vi "WSS.Generate.Digital.vi"(11 "Settings":T1={"ACTIVE EDGE"=TRUE, "ACTIVE TICKS"=0, "INACTIVE TICKS"=0, "DATA"=0, "SENSOR TYPE"=0}) -> (1 "Bit1":bool, 2 "Bit0":bool, 3 "Pulse":bool)   [LabVIEW 2018, in "Speciality FPGA IO.lvlib"]
doc: "This VI Simulates Wheel Speed Sensors for Unidirectional, Bidirectional - Bosch, and Bidirectional Conti. Sensor Type is:\n0 - Unidirectional\n1 - Bidirectional Bosch\n2 - Bidirectional Continental. The output of the VI is two digital bits that correspond to the following current levels when paired with an OW-902 module:\nBit 0 Bit 1 Output Current Level\n0 0 0\n0 1 Lo\n1 0 Mid\n1 1 Hi"
uses:
  <vilib>/NI/FPGA Addon Specialty IO/Speciality FPGA IO.lvlib
  <vilib>/NI/FPGA Addon Specialty IO/Types/WSS.Generate.Digital.Settings.ctl
  <vilib>/NI/FPGA Addon Specialty IO/Types/PWM.Generate.Digital.Settings.ctl
  <vilib>/NI/FPGA Addon Specialty IO/Types/WSS.Sensor.Type.ctl
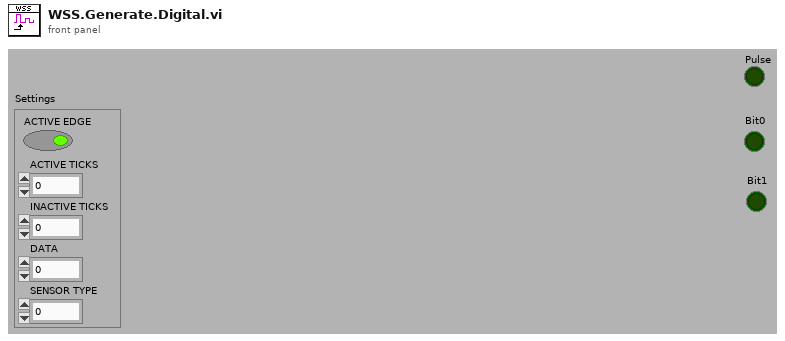
[diagram p1: front panel]
types:
  T1 = typedef "Speciality FPGA IO.lvlib/WSS.Generate.Digital.Settings.ctl" = cluster{"ACTIVE EDGE":bool, "ACTIVE TICKS":u32, "INACTIVE TICKS":u32, "DATA":u8, "SENSOR TYPE":u8}
  T2 = typedef "Speciality FPGA IO.lvlib/PWM.Generate.Digital.Settings.ctl" = cluster{"ACTIVE EDGE":bool, "ACTIVE TICKS":u32, "INACTIVE TICKS":u32}
  T3 = typedef "Speciality FPGA IO.lvlib/WSS.Sensor.Type.ctl" = enum16{"Unidirectional", "Bosch Bidirectional", "Continental Bidirectional"}
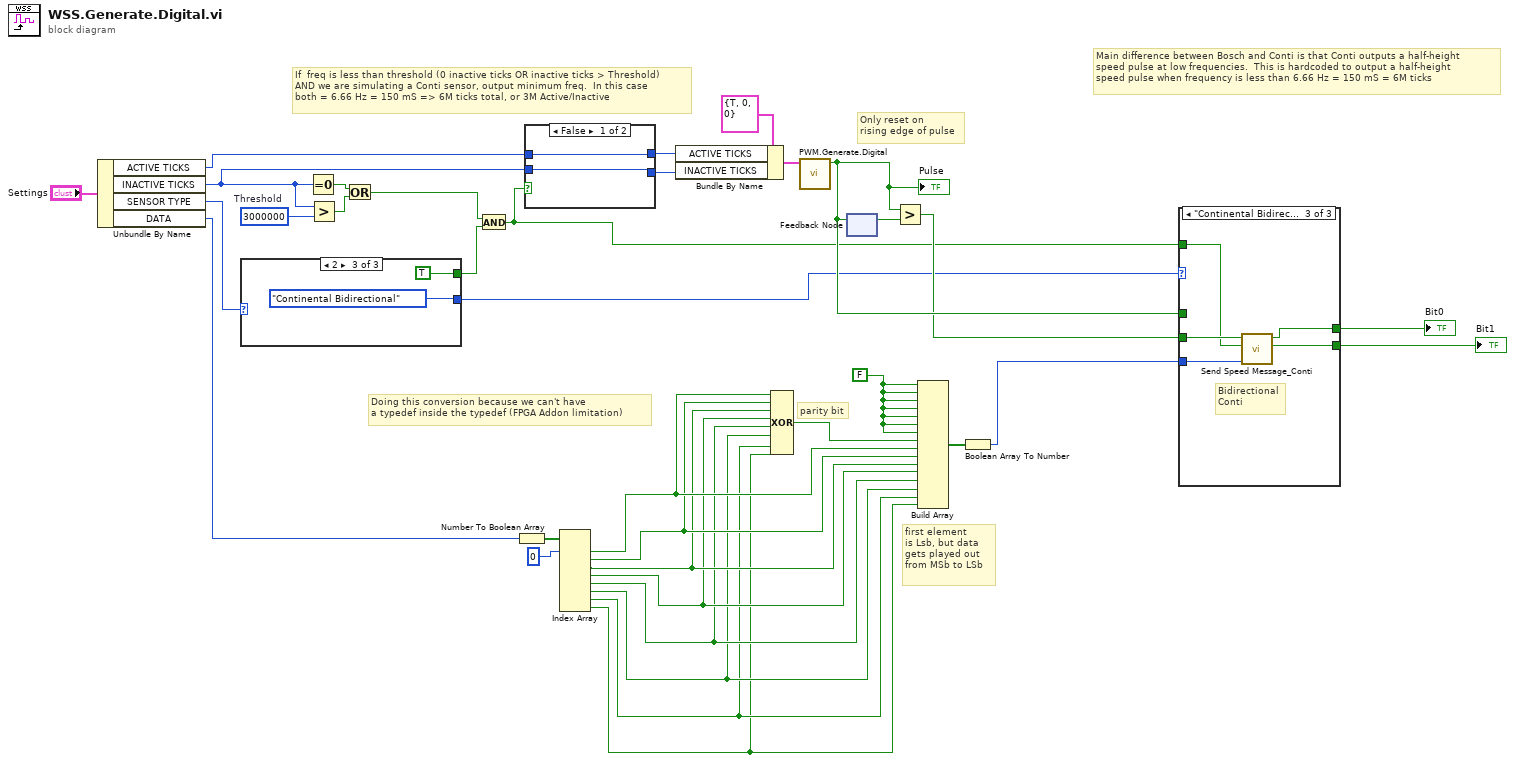
[diagram p0: block diagram]
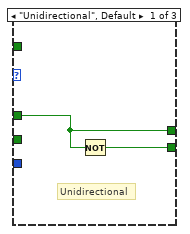
[diagram p2: hidden frame]
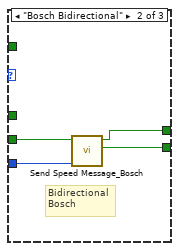
[diagram p3: hidden frame]
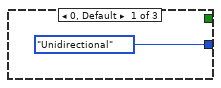
[diagram p4: hidden frame]
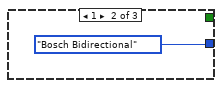
[diagram p5: hidden frame]
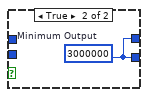
[diagram p6: hidden frame]
diagram:
  w20 = u32 3000000  # Threshold
  w33 = FALSE ("element")
  # "Doing this conversion because we can't have\na typedef inside the typedef (FPGA Addon limitation)"
  # "first element\nis Lsb, but data \ngets played out \nfrom MSb to LSb"
  # "Only reset on\nrising edge of pulse"
  # "If  freq is less than threshold (0 inactive ticks OR inactive ticks > Threshold) \nAND we are simulating a Conti sensor, output minimum freq.  In this case \nboth = 6.66 Hz = 150 mS => 6M ticks total, or 3M Active/Inactive"
  # "Main difference between Bosch and Conti is that Conti outputs a half-height\nspeed pulse at low frequencies.  This is hardcoded to output a half-height\nspeed pulse when frequency is less than 6.66 Hz = 150 mS = 6M ticks"
  # "parity bit"
  n1 = Unbundle By Name("Settings") -> ("ACTIVE TICKS"=w9:u32, "INACTIVE TICKS"=w8:u32, "SENSOR TYPE"=w3:u8, "DATA"=w16:u8)
  n2 = case shown="2" w3 {
    tunnel: [WSS.Sensor.Type."Unidirectional" ("Sensor Type") WSS.Sensor.Type."Bosch Bidirectional" ("Sensor Type") WSS.Sensor.Type."Continental Bidirectional" ("Sensor Type")] -> w2
    tunnel: [_ _ TRUE] -> w1
    frame 0, Default {
    }
    frame 1 {
    }
    frame 2 {
    }
  }
  n3 = Equal To 0?(x=w8) -> (x = 0?=w13:bool)
  n4 = Greater?(x=w8, y=w20) -> (0:w12:bool)
  n5 = Or(x=w13, y=w12) -> (x .or. y?=w11:bool)
  n6 = And(x=w11, y=w1) -> (x .and. y?=w10:bool)
  n7 = Number To Boolean Array(number=w16) -> (Boolean array=w30:bool[])
  n8 = case shown="False" w10 {
    tunnel: [w40 w42] -> w7
    tunnel: [w41 w42] -> w6
    tunnel: w9 -> [w41 _]
    tunnel: w8 -> [w40 _]
    frame False {
    }
    frame True {
      w42 = u32 3000000  # Minimum Output
    }
  }
  n9 = Index Array(array=w30, index #1=0 ("index")) -> (element #1=w28:bool, element #2=w27:bool, element #3=w26:bool, element #4=w25:bool, element #5=w24:bool, element #6=w23:bool, element #7=w22:bool, element #8=w21:bool)  [unwired: 7 in]
  n10 = Bundle By Name(cluster=T2 {"ACTIVE EDGE"=TRUE, "ACTIVE TICKS"=0, "INACTIVE TICKS"=0} ("Settings"), "ACTIVE TICKS"=w6, "INACTIVE TICKS"=w7) -> (w14:T2)
  n11 = Compound Arithmetic op=XOR(w28, w27, w26, w25, w24, w23, w22, w21) -> (w31:bool)
  n12 = call <vilib>:"PWM.Generate.Digital.vi"("Settings"=w14) -> ("Output"=w19:bool)  [unwired: 10 in]
  "Pulse" <- w19
  n13 = feedback #1() -> (w32:bool)  [unwired: 1 in]
  n14 = feedback-in #1(w19) -> ()
  n15 = Greater?(x=w19, y=w32) -> (0:w18:bool)
  n16 = Build Array(w33, w33, w33, w33, w33, w33, w33, w31, w28, w27, w26, w25, w24, w23, w22, w21) -> (w35:bool[])
  n17 = Boolean Array To Number(Boolean array=w35) -> (number=w34:u16)
  n18 = case shown="\"Continental Bidirectional\"" w2 {
    tunnel: w34 -> [_ w48 w53]
    tunnel: w18 -> [_ w47 w52]
    tunnel: [w43 w46 w51] -> w5
    tunnel: [w44 w45 w50] -> w4
    tunnel: w19 -> [w43 _ _]
    tunnel: w10 -> [_ _ w49]
    frame "Unidirectional", Default {
      # "Unidirectional"
      n19 = Not(x=w43) -> (.not. x?=w44:bool)
    }
    frame "Bosch Bidirectional" {
      # "Bidirectional\nBosch"
      n20 = call <vilib>:"Send Speed Message_Bosch.vi"("Data"=w48, "Reset"=w47) -> ("Bit 1 Out"=w45:bool, "Bit 0 Out"=w46:bool)  [unwired: 6 in]
    }
    frame "Continental Bidirectional" {
      # "Bidirectional\nConti"
      n21 = call <vilib>:"Send Speed Message_Conti.vi"("Data"=w53, "Standstill"=w49, "Reset"=w52) -> ("Bit 1 Out"=w50:bool, "Bit 0 Out"=w51:bool)  [unwired: 5 in]
    }
  }
  "Bit0" <- w5
  "Bit1" <- w4
